vi "B Spline.vi"(6 "percision":dbl=0.01, 7 "weights":dbl[](array[numeric]), 8 "error in":errorcluster, 9 "knots":dbl[](array[numeric]), 10 "degree":u16, 11 "points":dbl[][](array[numeric])) -> (0 "error out":errorcluster, 3 "spline":dbl[][](array[numeric]))   [LabVIEW 2019]
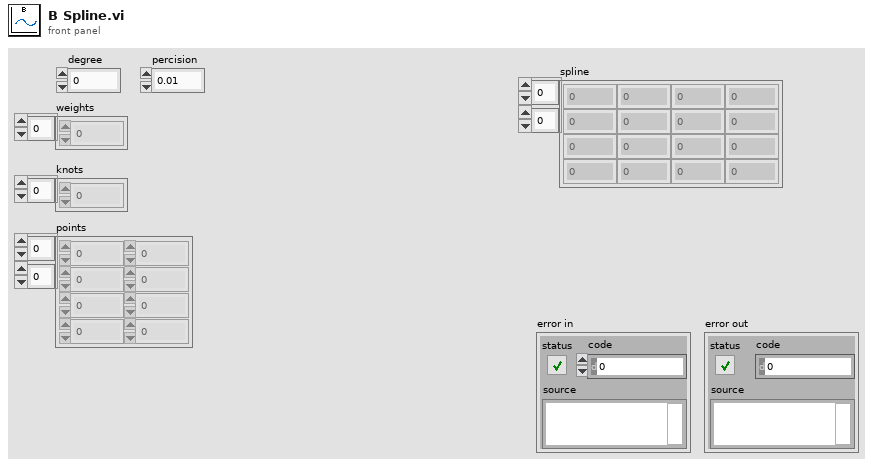
[diagram p1: front panel]
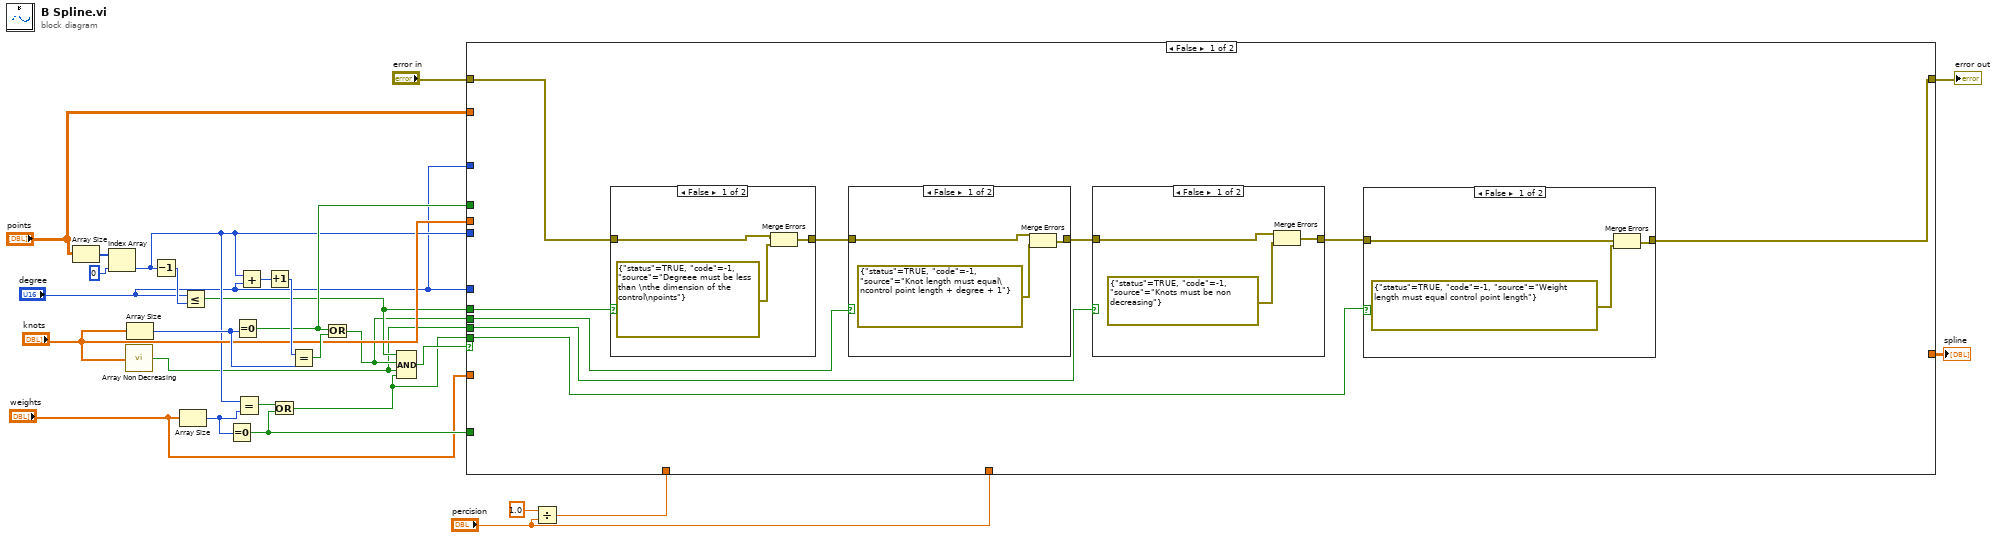
[diagram p0: block diagram]
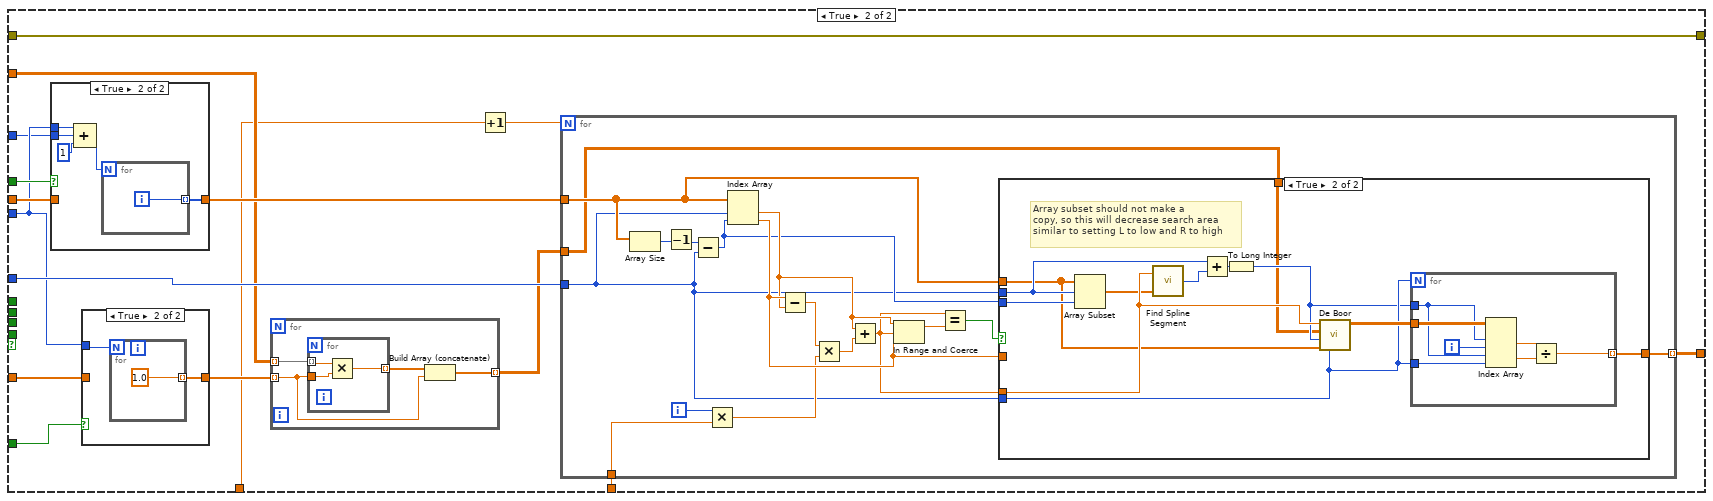
[diagram p6: hidden frame]
diagram:
  n1 = Array Size(array="points") -> (size(s)=w12:i32[])
  n2 = Index Array(array=w12, index=0) -> (element=w11:i32)
  n3 = call "Array Non Decreasing.vi"("array"="knots") -> ("Non Decreasing?"=w2:bool)
  n4 = Array Size(array="knots") -> (size(s)=w19:i32)
  n5 = Decrement(x=w11) -> (x-1=w27:i32)
  n6 = Array Size(array="weights") -> (size(s)=w22:i32)
  n7 = Less Or Equal?(x="degree", y=w27) -> (x <= y?=w4:bool)
  n8 = Equal To 0?(x=w22) -> (x = 0?=w21:bool)
  n9 = Equal To 0?(x=w19) -> (x = 0?=w18:bool)
  n10 = Equal?(x=w11, y=w22) -> (x = y?=w23:bool)
  n11 = Add(x=w11, y="degree") -> (x+y=w25:i32)
  n12 = Increment(x=w25) -> (x+1=w24:i32)
  n13 = Or(x=w23, y=w21) -> (x .or. y?=w1:bool)
  n14 = Equal?(x=w24, y=w19) -> (x = y?=w20:bool)
  n15 = Or(x=w18, y=w20) -> (x .or. y?=w3:bool)
  n16 = Compound Arithmetic op=AND(w4, w3, w2, w1) -> (w26:bool)
  n17 = Divide(x=1.0, y="percision") -> (x/y=w15:dbl)
  n18 = case shown="False" w26 {
    tunnel: w21 -> [_ w68]
    tunnel: "weights" -> [_ w67]
    tunnel: w11 -> [_ w60]
    tunnel: w18 -> [_ w66]
    tunnel: "knots" -> [_ w65]
    tunnel: "points" -> [_ w57]
    tunnel: "degree" -> [_ w63]
    tunnel: w15 -> [_ w54]
    tunnel: "percision" -> [_ w62]
    tunnel: "degree" -> [_ w59]
    tunnel: [_ w58] -> w7
    tunnel: "error in" -> [w35 w53]
    tunnel: [w28 w53] -> w5
    tunnel: w4 -> [w36 _]
    tunnel: w3 -> [w33 _]
    tunnel: w2 -> [w31 _]
    tunnel: w1 -> [w29 _]
    frame False {
      n19 = case shown="False" w36 {
        tunnel: [w51 w52] -> w34
        tunnel: w35 -> [w50 w52]
        frame False {
          n20 = Merge Errors(w50, errorcluster {"status"=TRUE, "code"=-1, "source"="Degreee must be less than \nthe dimension of the control\npoints"} ("error constant")) -> (w51:errorcluster)
        }
        frame True {
        }
      }
      n21 = case shown="False" w33 {
        tunnel: [w45 w48] -> w32
        tunnel: w34 -> [w46 w48]
        frame False {
          n22 = Merge Errors(w46, errorcluster {"status"=TRUE, "code"=-1, "source"="Knot length must equal\ncontrol point length + degree + 1"} ("error constant")) -> (w45:errorcluster)
        }
        frame True {
        }
      }
      n23 = case shown="False" w31 {
        tunnel: [w41 w44] -> w30
        tunnel: w32 -> [w42 w44]
        frame False {
          n24 = Merge Errors(w42, errorcluster {"status"=TRUE, "code"=-1, "source"="Knots must be non decreasing"} ("error constant")) -> (w41:errorcluster)
        }
        frame True {
        }
      }
      n25 = case shown="False" w29 {
        tunnel: [w37 w40] -> w28
        tunnel: w30 -> [w39 w40]
        frame False {
          n26 = Merge Errors(w39, errorcluster {"status"=TRUE, "code"=-1, "source"="Weight length must equal control point length"} ("error constant")) -> (w37:errorcluster)
        }
        frame True {
        }
      }
    }
    frame True {
      n27 = case shown="True" w66 {
        tunnel: w65 -> [w76 _]
        tunnel: [w76 w81] -> w64
        tunnel: w60 -> [_ w80]
        tunnel: w59 -> [_ w79]
        frame False {
        }
        frame True {
          n28 = Compound Arithmetic op=ADD(w80, w79, u16 1 ("value")) -> (w77:i32)
          n29 = for {
            N: w77 -> [_]
            tunnel: [w82] -> w81 mode=indexing
            i -> [w82]
          }
        }
      }
      n30 = case shown="True" w68 {
        tunnel: w67 -> [w83 _]
        tunnel: [w83 w84] -> w55
        tunnel: w60 -> [_ w85]
        frame False {
        }
        frame True {
          n31 = for {
            N: w85 -> [_]
            tunnel: [1.0] -> w84 mode=indexing
          }
        }
      }
      n32 = for {
        tunnel: w57 -> [w72] mode=indexing
        tunnel: w55 -> [w70] mode=indexing
        tunnel: [w69] -> w56 mode=indexing
        n33 = for {
          tunnel: w72 -> [w75] mode=indexing
          tunnel: w70 -> [w74]
          tunnel: [w73] -> w71 mode=indexing
          n34 = Multiply(x=w75, y=w74) -> (x*y=w73:dbl)
        }
        n35 = Build Array (concatenate)(w71, w70) -> (w69:dbl[])
      }
      n36 = Increment(x=w54) -> (x+1=w61:dbl)
      n37 = for {
        N: w61 -> [_]
        tunnel: w64 -> [w98]
        tunnel: w56 -> [w97]
        tunnel: w63 -> [w87]
        tunnel: w62 -> [w100]
        tunnel: [w96] -> w58 mode=indexing
        i -> [w101]
        n38 = Array Size(array=w98) -> (size(s)=w103:i32)
        n39 = Decrement(x=w103) -> (x-1=w102:i32)
        n40 = Subtract(x=w102, y=w87) -> (x-y=w88:i32)
        n41 = Multiply(x=w101, y=w100) -> (x*y=w91:dbl)
        n42 = Index Array(array=w98, index #1=w87, index #2=w88) -> (element #1=w94:dbl, element #2=w95:dbl)
        n43 = Subtract(x=w95, y=w94) -> (x-y=w89:dbl)
        n44 = Multiply(x=w89, y=w91) -> (x*y=w99:dbl)
        n45 = Add(x=w94, y=w99) -> (x+y=w90:dbl)
        n46 = In Range and Coerce(upper limit=w94, x=w90, lower limit=w95) -> (coerced(x)=w93:dbl)  [unwired: 1 out]
        n47 = Equal?(x=w90, y=w93) -> (x = y?=w92:bool)
        n48 = case shown="True" w92 {
          tunnel: w98 -> [_ w104]
          tunnel: w95 -> [_ _]
          tunnel: w90 -> [_ w115]
          tunnel: w97 -> [_ w105]
          tunnel: w87 -> [_ w113]
          tunnel: [_ w112] -> w96
          tunnel: w88 -> [_ w110]
          tunnel: w87 -> [_ w106]
          frame False {
          }
          frame True {
            # "Array subset should not make a\ncopy, so this will decrease search area\nsimilar to setting L to low and R to high"
            n49 = Array Subset(array=w104, index=w106, length=w110) -> (w111:dbl[])
            n50 = call "Find Spline Segment.vi"("knots"=w111, "position"=w115) -> ("spline segment idx"=w109:i32)
            n51 = Add(x=w106, y=w109) -> (x+y=w108:i32)
            n52 = To Long Integer(number=w108) -> (32bit integer=w107:i32)
            n53 = call "De Boor.vi"("degree"=w113, "knots"=w104, "spline segment idx"=w107, "points"=w105, "position"=w115) -> ("points out"=w114:dbl[][])  [unwired: 6 in]
            n54 = for {
              N: w113 -> [_]
              tunnel: w114 -> [w122]
              tunnel: w107 -> [w120]
              tunnel: w113 -> [w119]
              tunnel: [w116] -> w112 mode=indexing
              i -> [w121]
              n55 = Index Array(array=w122, index (row) #1=w120, index (col) #1=w121, index (row) #2=w120, index (col) #2=w119) -> (element #1=w117:dbl, element #2=w118:dbl)
              n56 = Divide(x=w117, y=w118) -> (x/y=w116:dbl)
            }
          }
        }
      }
    }
  }
  "error out" <- w5
  "spline" <- w7
